vi "Init.vi"(8 "error in (no error)":errorcluster, 11 "Debug":bool) -> (0 "error out":errorcluster, 3 "BadRequestException out":refnum<class "BadRequestException.lvclass">)   [LabVIEW 2020, in "HTTP Server.lvlib" / "BadRequestException.lvclass"]
uses:
  BadRequestException.lvclass
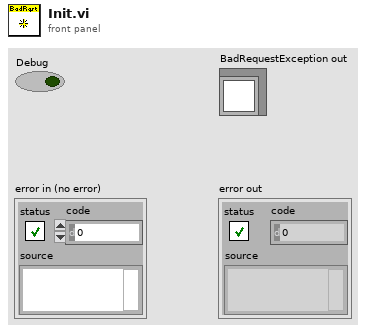
[diagram p1: front panel]
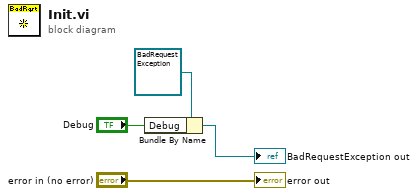
[diagram p0: block diagram]
diagram:
  n1 = Bundle By Name(cluster=refnum<class "BadRequestException.lvclass"> refnum ("BadRequestException in"), "Debug"="Debug") -> (→"BadRequestException out":refnum<class "BadRequestException.lvclass">)
  "error out" <- "error in (no error)"
